vi "VisionTurnSmooth.vi"(5 "Min Power":dbl, 6 "First Time?":bool, 7 "Target Range":dbl, 8 "Current Position":dbl, 9 "Target Position":dbl, 10 "Slow Range":dbl, 11 "Motor Power In":dbl) -> (0 "Done":bool, 2 "Right Motor Power":dbl, 3 "Left Motor Power":dbl)   [LabVIEW 2016]
panel:
  out "Speed Closed Loop Plots":cluster{dbl, "Sensor Velocity":dbl}(graph)
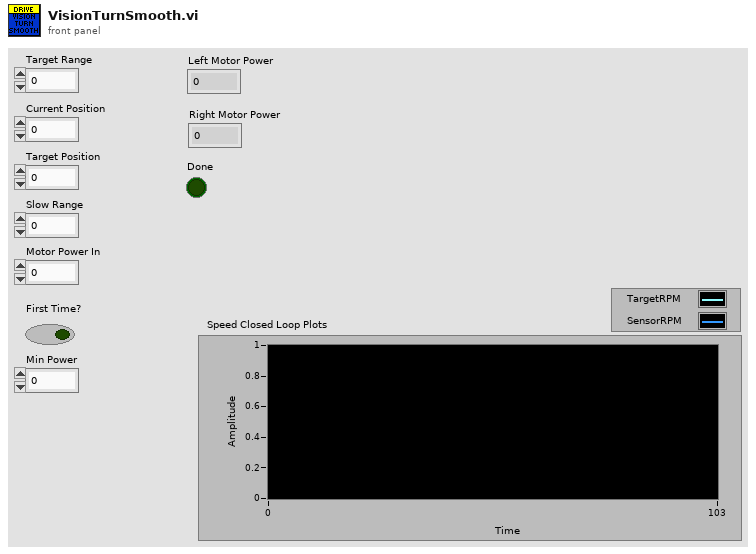
[diagram p1: front panel]
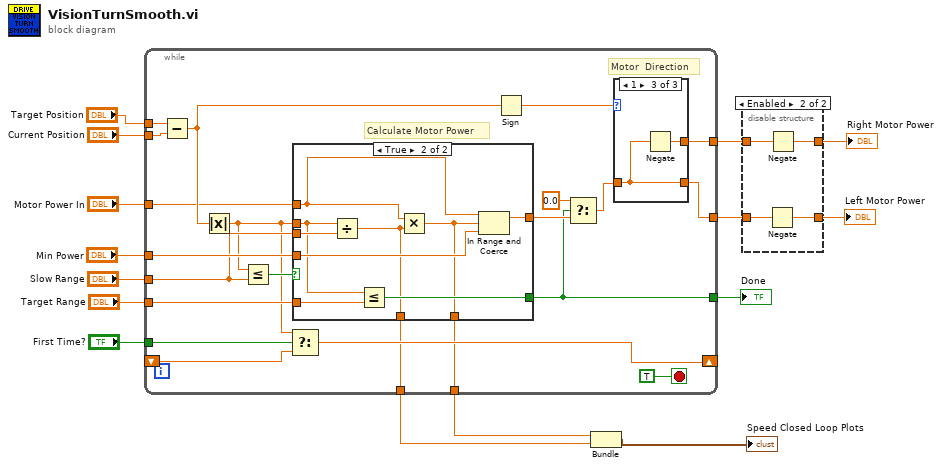
[diagram p0: block diagram]
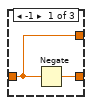
[diagram p3: hidden frame]
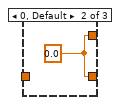
[diagram p4: hidden frame]
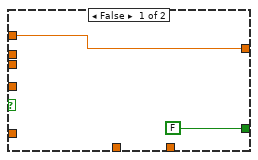
[diagram p5: hidden frame]
diagram:
  n1 = while {
    shift-right: [w35] -> _
    shift-left: _ -> [w36]
    tunnel: [w23] -> w15
    tunnel: [w31] -> w7
    tunnel: [w30] -> w5
    tunnel: "Current Position" -> [w20]
    tunnel: "Target Position" -> [w19]
    tunnel: "Motor Power In" -> [w29]
    tunnel: "Min Power" -> [w28]
    tunnel: "Slow Range" -> [w21]
    tunnel: "Target Range" -> [w27]
    tunnel: "First Time?" -> [w26]
    tunnel: [w17] -> w2
    tunnel: [w16] -> w1
    stop <- TRUE stop-if-true
    # "Motor  Direction"
    # "Calculate Motor Power"
    n2 = Subtract(x=w19, y=w20) -> (x-y=w33:dbl)
    n3 = Absolute Value(x=w33) -> (abs(x)=w18:dbl)
    n4 = Less Or Equal?(x=w18, y=w21) -> (x <= y?=w34:bool)
    n5 = Select(t=w18, s=w26, f=w36) -> (s? t:f=w35:dbl)
    n6 = case shown="True" w34 {
      tunnel: w18 -> [_ w45]
      tunnel: w27 -> [_ w51]
      tunnel: [FALSE w49] -> w23
      tunnel: [w43 w53] -> w25
      tunnel: w29 -> [w43 w52]
      tunnel: w28 -> [_ w50]
      tunnel: w21 -> [_ w48]
      tunnel: [_ w46] -> w17
      tunnel: [_ w47] -> w16
      frame False {
      }
      frame True {
        n7 = Divide(x=w45, y=w48) -> (x/y=w46:dbl)
        n8 = Less Or Equal?(x=w45, y=w51) -> (x <= y?=w49:bool)
        n9 = Multiply(x=w52, y=w46) -> (x*y=w47:dbl)
        n10 = In Range and Coerce(upper limit=w52, x=w47, lower limit=w50) -> (coerced(x)=w53:dbl)  [unwired: 1 out]
      }
    }
    n11 = Sign(1:w33) -> (0:w32:dbl)
    n12 = Select(t=0.0, s=w23, f=w25) -> (s? t:f=w24:dbl)
    n13 = case shown="1" w32 {
      tunnel: [w39 w40 w41] -> w31
      tunnel: [w38 w40 w42] -> w30
      tunnel: w24 -> [w38 _ w41]
      frame -1 {
        n14 = Negate(x=w38) -> (-x=w39:dbl)
      }
      frame 0, Default {
        w40 = 0.0
      }
      frame 1 {
        n15 = Negate(x=w41) -> (-x=w42:dbl)
      }
    }
  }
  "Done" <- w15
  n16 = Bundle(w1, w2) -> (→"Speed Closed Loop Plots":cluster{dbl, dbl})  [unwired: 1 in]
  n17 = disable-structure shown="Enabled" {
    disable-tunnel: w7 -> [w55 w59]
    disable-tunnel: [w55 w58] -> w6
    disable-tunnel: w5 -> [w54 w57]
    disable-tunnel: [w54 w56] -> w4
    frame Disabled {
    }
    frame Enabled {
      n18 = Negate(x=w59) -> (-x=w58:dbl)
      n19 = Negate(x=w57) -> (-x=w56:dbl)
    }
  }
  "Left Motor Power" <- w6
  "Right Motor Power" <- w4
